vi "exnSpectralBlock spectral measurements RMS WFM (CDB).vi"(0 "Signals":waveform(cdb), 5 "Restart Averaging":bool, 7 "View":T2, 9 "Spectrum Window":u16, 11 "error in (no error)":errorcluster, 12 "Spectrum Averaging Parameters":T1={"averaging mode"=0, "weighting mode"=1, "number of averages"=10} {"averaging mode" items=["No averaging", "Vector averaging", "RMS averaging", "Peak hold"]; "weighting mode" items=["Linear", "Exponential"]}, 14 "All Spectra":bool) -> (4 "Measurement Output":cluster{"f0":dbl, "df":dbl, "magnitude":dbl[]}(graph), 6 "averaging done":bool, 10 "Phase":cluster{"f0":dbl, "df":dbl, "phase":dbl[]}(graph), 15 "error out":errorcluster)   [LabVIEW 2020]
uses:
  <vilib>/measure/NI_MAPro.lvlib
panel:
  in  "measurement":string="FFT - (RMS)"
  in  "string":string=" Phase"
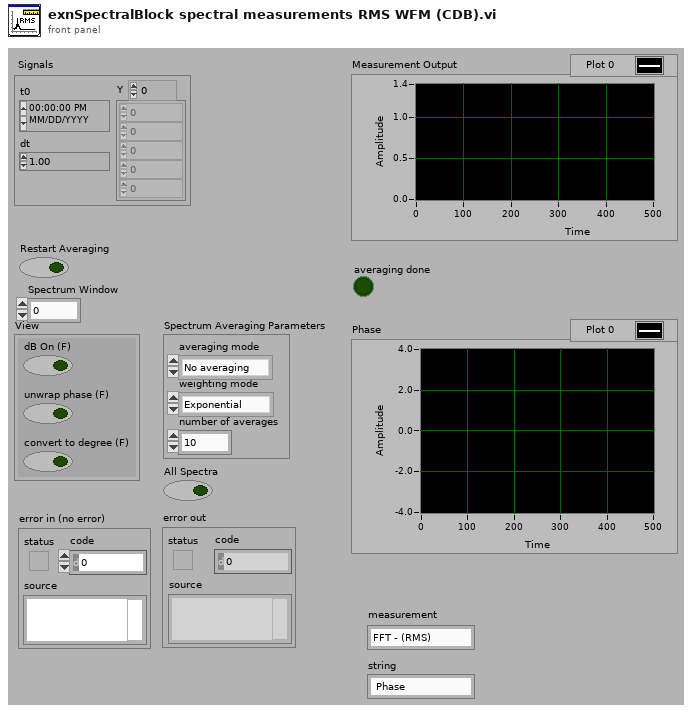
[diagram p1: front panel]
types:
  T1 = cluster{"averaging mode":u16, "weighting mode":u16, "number of averages":u32}
  T2 = cluster{"dB On (F)":bool, "unwrap phase (F)":bool, "convert to degree (F)":bool}
  T3 = enum16{"None ", "Hanning", "Hamming", "Blackman-Harris", "Exact Blackman", "Blackman", "Flat Top", "4 Term B-Harris ", "7 Term B-Harris", "Low Sidelobe"}
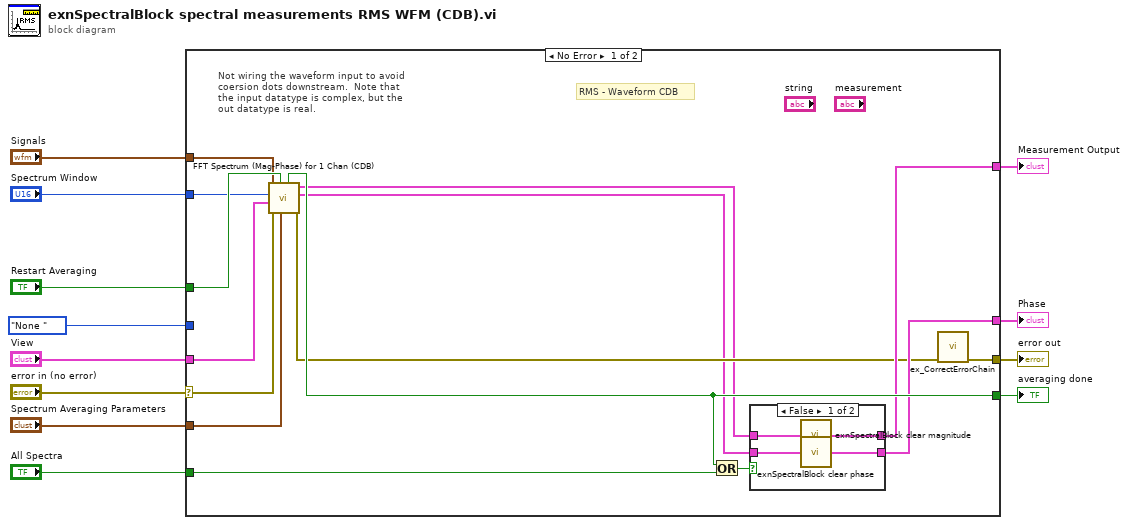
[diagram p0: block diagram]
diagram:
  n1 = case shown="No Error" "error in (no error)" {
    selector: "error in (no error)" -> [w19 w34]
    tunnel: [w18 _] -> w12
    tunnel: [w17 _] -> w11
    tunnel: [w27 _] -> w10
    tunnel: "All Spectra" -> [w26 _]
    tunnel: "Spectrum Averaging Parameters" -> [w25 _]
    tunnel: "Restart Averaging" -> [w24 _]
    tunnel: T3."None " ("window") -> [_ _]
    tunnel: "Spectrum Window" -> [w20 _]
    tunnel: "View" -> [w23 _]
    tunnel: "Signals" -> [w13 _]
    tunnel: [w22 w34] -> w4
    frame No Error {
      # "Not wiring the waveform input to avoid coersion dots downstream.  Note that the input datatype is complex, but the out datatype is real."
      # "RMS - Waveform CDB"
      n2 = call <vilib>:"FFT Spectrum (Mag-Phase) for 1 Chan (CDB).vi"("averaging parameters"=w25, "restart averaging (F)"=w24, "error in (no error)"=w19, "view"=w23, "window"=w20, "time signal"=w13) -> ("error out"=w16:errorcluster, "phase"=w14:cluster{"f0":dbl, "df":dbl, "phase":dbl[]}, "magnitude"=w15:cluster{"f0":dbl, "df":dbl, "magnitude":dbl[]}, "averaging done"=w27:bool)  [unwired: 1 in, 1 out]
      n3 = Or(x=w27, y=w26) -> (x .or. y?=w21:bool)
      n4 = case shown="False" w21 {
        tunnel: w14 -> [w29 w32]
        tunnel: w15 -> [w31 w33]
        tunnel: [w30 w33] -> w18
        tunnel: [w28 w32] -> w17
        frame False {
          n5 = call <vilib>:"exnSpectralBlock clear magnitude.vi"("magnitude in"=w31) -> ("magnitude out"=w30:cluster{"f0":dbl, "df":dbl, "magnitude":dbl[]})
          n6 = call <vilib>:"exnSpectralBlock clear phase.vi"("phase in"=w29) -> ("phase out"=w28:cluster{"f0":dbl, "df":dbl, "phase":dbl[]})
        }
        frame True {
        }
      }
      n7 = call <vilib>:"ex_CorrectErrorChain.vi"("error in (no error)"=w16) -> ("error out"=w22:errorcluster)  [unwired: 10 in]
    }
    frame Error {
    }
  }
  "Phase" <- w11
  "Measurement Output" <- w12
  "averaging done" <- w10
  "error out" <- w4
